vi "Configure DANL Measurement.vi"(0 "VISA resource name":refnum<visa-resource-name>, 5 "DANL Measurement Method (0: Attenuator)":i32(ring) items=["Attenuator", "Removal"], 7 "DANL Cancellation Deviation Threshold (2.5 dB)":dbl=2.5, 9 "DANL Cancellation Reference Trace (1: Trace 1)":i32(ring)=1 items=["Trace 1"=1, "Trace 2"=2, "Trace 3"=3], 11 "error in (no error)":errorcluster) -> (4 "VISA resource name out":refnum<visa-resource-name>, 15 "error out":errorcluster)   [LabVIEW 2014, in "Agilent ESA PSA Series.lvlib"]
doc: "Configures the DANL cancellation settings for a log plot measurement with cancellation.\n\n<B>Note:</B> \n\nThis VI is only valid in Phase Noise personality. Use <B>Switch Personality</B> VI to switch to Phase Noise before calling this VI."
uses:
  Agilent ESA PSA Series.lvlib
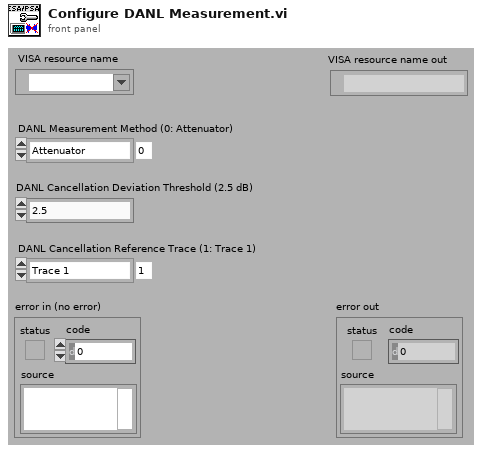
[diagram p1: front panel]
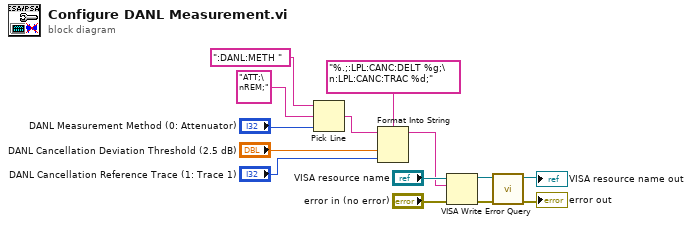
[diagram p0: block diagram]
diagram:
  n1 = Pick Line(string ("")=":DANL:METH " ("initial string"), multi-line string="ATT;\nREM;", line index="DANL Measurement Method (0: Attenuator)") -> (output string=w4:string)
  n2 = Format Into String(format string="%.;:LPL:CANC:DELT %g;\n:LPL:CANC:TRAC %d;", initial string=w4, "DANL Cancellation Deviation Threshold (2.5 dB)", "DANL Cancellation Reference Trace (1: Trace 1)") -> (resulting string=w1:string)  [unwired: 1 in, 1 out]
  n3 = VISA Write(VISA resource name="VISA resource name", write buffer=w1, error in (no error)="error in (no error)") -> (VISA resource name out=w10:refnum<visa-resource-name>, error out=w9:errorcluster)  [unwired: 1 out]
  n4 = call "Error Query.vi"("error in (no error)"=w9, "VISA resource name"=w10) -> ("error out"=→"error out":errorcluster, "VISA resource name out"=→"VISA resource name out":refnum<visa-resource-name>)  [unwired: 6 in, 2 out]
